vi "RQST Lookup Table Act.vi"(7 "Action":enum16{"Initialize", "Add", "Get", "Remove"}(ring), 8 "error in (no error)":errorcluster, 9 "ID":u32, 10 "Data":T1, 11 "ref in":T2) -> (0 "error out":errorcluster {"code" min=0 max=0}, 1 "Found?":bool, 2 "Data":T1)   [LabVIEW 2013, in "J1939 Addon Engine.lvlib"]
uses:
  Engine/J1939 Addon Engine.lvlib
  Types/RQST Lookup Table Reference.ctl
  Types/RQST Lookup Table Cluster.ctl
  <vilib>/xnet/xnet.llb/XNET Frame CAN.ctl
  <vilib>/xnet/xnet.llb/XNET Frame Type CAN.ctl
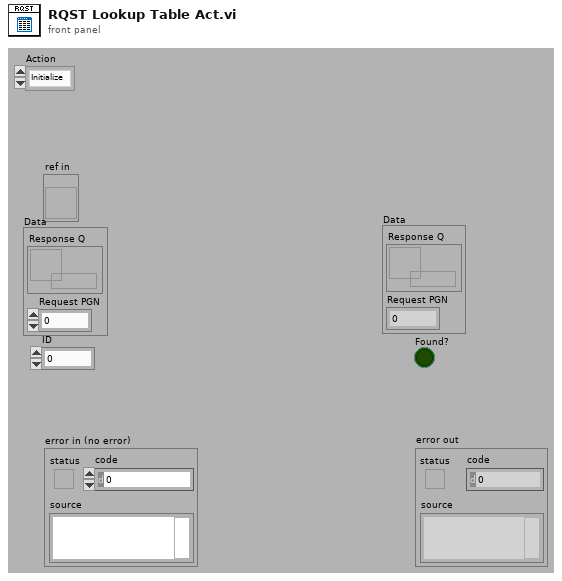
[diagram p1: front panel]
types:
  T1 = typedef "J1939 Addon Engine.lvlib/RQST Lookup Table Cluster.ctl" = cluster{"Response Q":refnum<queue>, "Request PGN":u32}
  T2 = typedef "J1939 Addon Engine.lvlib/RQST Lookup Table Reference.ctl" = refnum<vi>
  T3 = typedef "J1939_RQST FG Cluster.ctl" = cluster{"Processed Incoming":refnum<queue>, "Request PGN":u32}
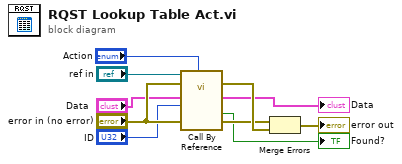
[diagram p0: block diagram]
diagram:
  n1 = call-by-ref "?"(reference="ref in", error in="error in (no error)", "Action"="Action", 8:"error in (no error)"="error in (no error)", "ID"="ID", "Data"="Data") -> (error out=w9:errorcluster, 0:"error out"=w6:errorcluster, "Found?"=→"Found?":bool, "Data Out"=→"Data":T3)  [unwired: 5 in, 1 out]
  n2 = Merge Errors(w6, w9) -> (→"error out":errorcluster)
